vi "Async.Engine.Initialize.vi"(6 "Timeout (ms) (5000)":u16=5000, 7 "Error Log Settings":T4, 8 "error in":errorcluster, 9 "Data Access Settings":T3 {"Read"."Refs"."Data Reference" format="%.0x"; "Write"."Refs" format="%.0x"; "ReadWrite"."Refs" format="%.0x"}, 10 "Processes":cluster{"VI":refnum<vi>, "Parameters":variant}[](array[cluster]), 11 "Name":string) -> (0 "error out":errorcluster, 3 "VS Plugin Inline Async API out":refnum<class "VS Plugin Inline Async API.lvclass">)   [LabVIEW 2024, in "VS Plugin Inline Async API.lvlib" / "VS Plugin Inline Async API.lvclass"]
uses:
  VS Plugin Inline Async API.lvclass
  VS Plugin Inline Async API.lvclass/VS Plugin Inline Async API.ctl
  Plugin Data Access Engine/Data Access Engine/Plugin Data Access Engine.lvclass
  Error Handling Process/Display and Log Process.vi
  VS Plugin Inline Async API.lvlib
  Types/Error Handling Settings.ctl
  <vilib>/NI VeriStand/Custom Device API/Data Reference.ctl
  <vilib>/NI VeriStand/Custom Device API/Custom Device API.lvlib
  <vilib>/NI VeriStand/Custom Device API/Block Data Reference.ctl
  VS Engine Abstraction/VS Engine Interface/VS Engine Interface.lvclass
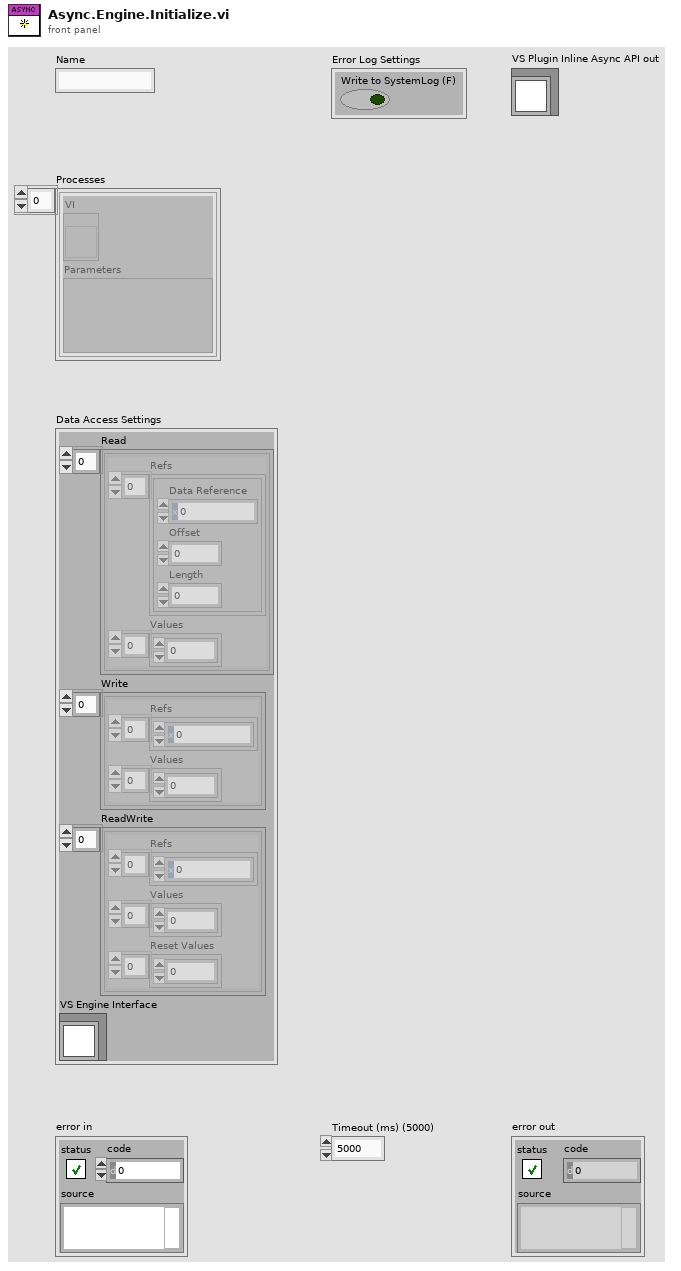
[diagram p1: front panel]
types:
  T1 = typedef "Custom Device API.lvlib/Block Data Reference.ctl" = cluster{"Data Reference":T2, "Offset":u64, "Length":u64}
  T2 = typedef "Custom Device API.lvlib/Data Reference.ctl" = i32
  T3 = cluster{"Read":cluster{"Refs":T1[], "Values":dbl[]}[], "Write":cluster{"Refs":T2[], "Values":dbl[]}[], "ReadWrite":cluster{"Refs":T2[], "Values":dbl[], "Reset Values":dbl[]}[], "VS Engine Interface":refnum<class "VS Engine Interface.lvclass">}
  T4 = typedef "VS Plugin Inline Async API.lvlib/VS Plugin Inline Async API.lvclass/Error Handling Settings.ctl" = cluster{"Write to SystemLog (F)":bool}
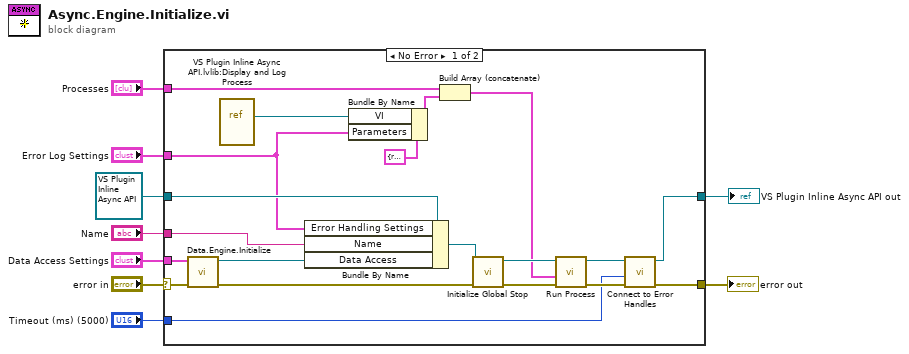
[diagram p0: block diagram]
diagram:
  n1 = case shown="No Error" "error in" {
    selector: "error in" -> [w26 w31]
    tunnel: [w28 w31] -> w8
    tunnel: [w21 w30] -> w4
    tunnel: refnum<class "VS Plugin Inline Async API.lvclass"> refnum ("VS Plugin Inline Async API out") -> [w24 w30]
    tunnel: "Processes" -> [w23 _]
    tunnel: "Error Log Settings" -> [w15 _]
    tunnel: "Timeout (ms) (5000)" -> [w14 _]
    tunnel: "Name" -> [w12 _]
    tunnel: "Data Access Settings" -> [w11 _]
    frame No Error {
      n2 = call "Data.Engine.Initialize.vi"("error in"=w26, "Data Access Settings"=w11) -> ("error out"=w25:errorcluster, "Data Access Engine"=w10:refnum<class "Plugin Data Access Engine.lvclass">)  [unwired: 8 in]
      n3 = vi-ref "VS Plugin Inline Async API.lvlib:Display and Log Process.vi"() -> (w13:refnum<vi>)
      n4 = Bundle By Name(cluster=w24, "Error Handling Settings"=w15, "Name"=w12, "Data Access"=w10) -> (w16:refnum<class "VS Plugin Inline Async API.lvclass">)
      n5 = Bundle By Name(cluster=cluster{"VI":refnum<vi>, "Parameters":variant} {"VI"=refnum, "Parameters"=variant} ("Process"), "VI"=w13, "Parameters"=w15) -> (w19:cluster{"VI":refnum<vi>, "Parameters":variant})
      n6 = Build Array (concatenate)(w23, w19) -> (w17:cluster{"VI":refnum<vi>, "Parameters":variant}[])
      n7 = call "Initialize Global Stop.vi"("error in"=w25, "VS Plugin Inline Async API in"=w16) -> ("error out"=w27:errorcluster, "VS Plugin Inline Async API out"=w18:refnum<class "VS Plugin Inline Async API.lvclass">)  [unwired: 8 in]
      n8 = call "Run Process.vi"("error in"=w27, "Processes"=w17, "VS Plugin Inline Async API in"=w18) -> ("error out"=w29:errorcluster, "VS Plugin Inline Async API out"=w22:refnum<class "VS Plugin Inline Async API.lvclass">)  [unwired: 7 in]
      n9 = call "Connect to Error Handles.vi"("error in"=w29, "Timeout (ms)"=w14, "VS Plugin Inline Async API in"=w22) -> ("error out"=w28:errorcluster, "VS Plugin Inline Async API out"=w21:refnum<class "VS Plugin Inline Async API.lvclass">)  [unwired: 7 in]
    }
    frame Error {
    }
  }
  "error out" <- w8
  "VS Plugin Inline Async API out" <- w4
